vi "send to debugview.vi"(6 "module":string, 7 "info type":T1(ring)=enum."Debug", 8 "error in":errorcluster, 11 "info":string) -> (0 "error out":errorcluster, 3 "string out":string)   [LabVIEW 2020, in "Reusable Library.lvlib"]
doc: "Send the information to windows built in diagnostic tool [System.Diagnostics.Debug] used for real time debugging. The information sent to this vi is not stored anywhere.\n\nUse Sysinternals DebugView application from Microsoft website to view the information."
uses:
  Reusable Library.lvlib
  kernel32.dll
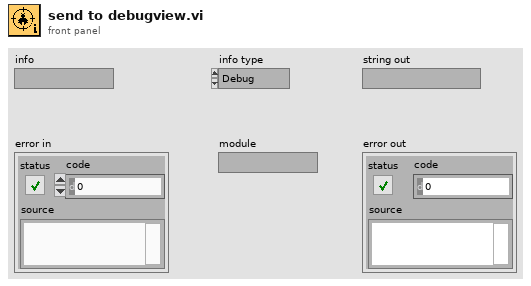
[diagram p1: front panel]
types:
  T1 = enum16{"Info", "Warning", "Error", "Debug", "Trace"}
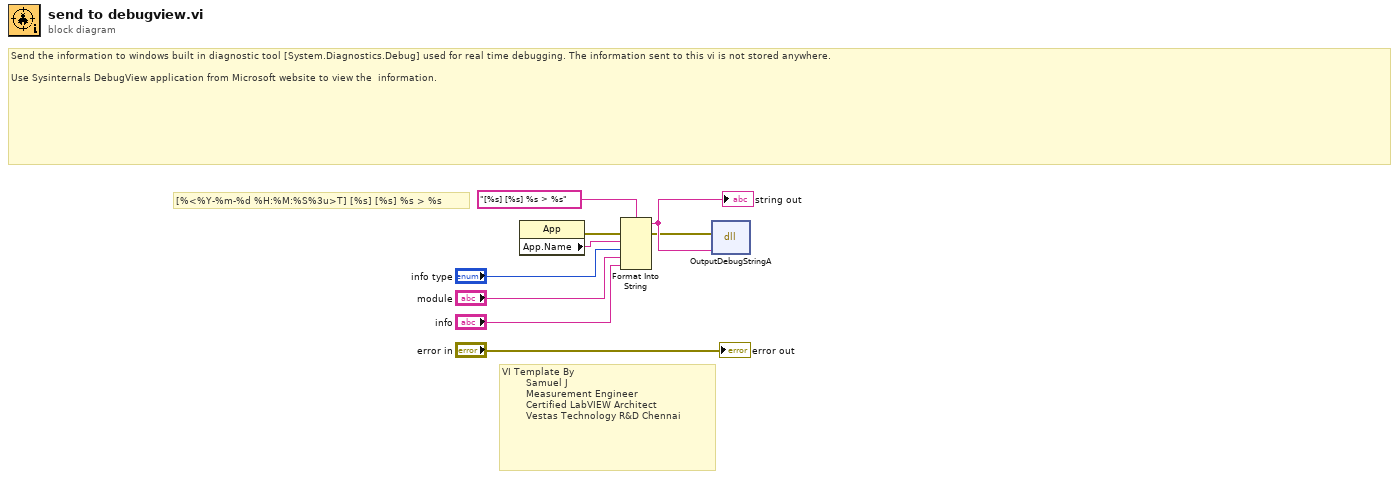
[diagram p0: block diagram]
diagram:
  # "Send the information to windows built in diagnostic tool [System.Diagnostics.Debug] used for real time debugging. The information sent to this vi is not stored anywhere.\n\nUse Sysinternals DebugView application from Microsoft website to view the  information."
  # "VI Template By\n        Samuel J\n        Measurement Engineer\n        Certified LabVIEW Architect\n        Vestas Technology R&D Chennai"
  # "[%<%Y-%m-%d %H:%M:%S%3u>T] [%s] [%s] %s > %s"
  n1 = property class="App"() -> (error out=w3:errorcluster, "App.Name"=w7:string)  [unwired: 2 in, 1 out]
  n2 = Format Into String(format string="[%s] [%s] %s > %s", error in=w3, w7, "info type", "module", "info") -> (resulting string=w4:string, error out=w2:errorcluster)  [unwired: 1 in]
  "string out" <- w4
  n3 = dll-call lib="kernel32.dll" fn="OutputDebugStringA"(error in=w2, "lpOutputString"=w4) -> ()  [unwired: 4 in, 2 out]
  "error out" <- "error in"
